vi "Recall Operating Mode.vi"(3 "error in":errorcluster, 4 "p1":i8, 5 "COM Port in":refnum<visa-resource-name>) -> (0 "error out":errorcluster, 1 "OK":bool, 2 "COM Port out":refnum<visa-resource-name>)   [LabVIEW 2013]
doc: "This command sets some bits of the operating mode through indexed presets.\n(Operating and bias level release, ACC/APC, analog/digital input releases and ICG activation)\n\nValid values for the parameter “p1” with PhoxX® lasers are:\no “0”: emission standby (the diode current source is set to 0)\no “1”: cw only – no modulation active\no “2”: digital modulated\no “3”: analog modulated\no “4”: digital and analog modulated\nAll other values will be refused.\n\nValid values for the parameter “p1” with LuxX® lasers are:\no “0”: emission standby (the diode current source is set to 0)\no “1”: ACC mode – no modulation active\no “2”: APC mode – no modulation active\no “3”: ACC mode – analog modulated\nAll other values will be refused.\n\nValid values for the parameter “p1” with LuxX+® and BrixX® lasers are:\no “0”: emission standby (the diode current source is set to 0)\no “1”: ACC mode – no modulation active\no “2”: APC mode – no modulation active\no “3”: ACC mode – digital modulated\no “4”: ACC mode – analog modulated\no “5”: ACC mode – digital and analog modulated\nAll other values will be refused.\n\nValid values for the parameter “p1” with LEDMOD.v2 are:\no “0”: emission standby (the diode current source is set to 0)\no “1”: cw only – no modulation active\no “2”: digital modulated\no “3”: analog modulated\no “4”: digital and analog modulated\no “5”: Internally PWM modulated - internal clock generator active (ICG)\no “6”: Internally PWM modulated - gated by external digital input\no “7”: Internally PWM modulated - externally modulated by analog input\no “8”: Internally PWM modulated - gated by digital input + externally modulated by analog input\nAll other values will be refused."
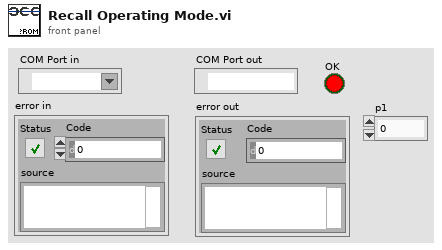
[diagram p1: front panel]
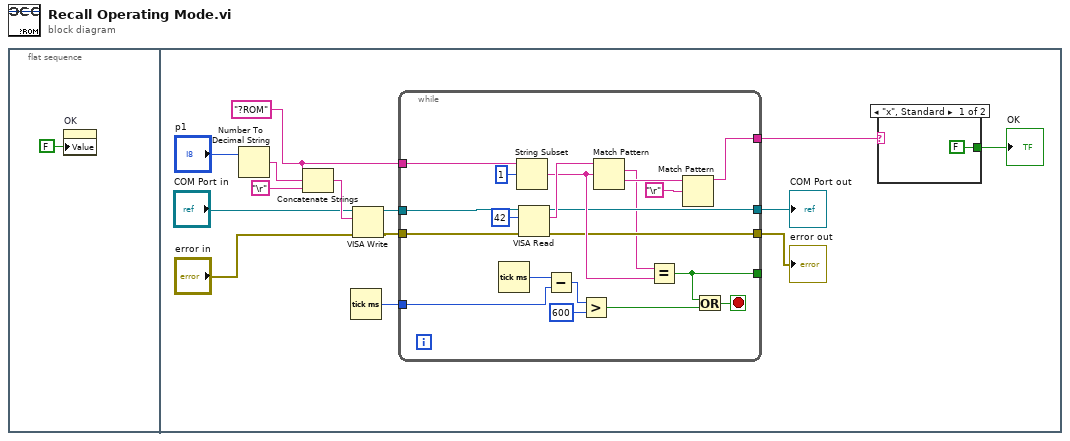
[diagram p0: block diagram]
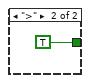
[diagram p2: hidden frame]
diagram:
  n1 = flat-sequence {
    frame #0 {
      n2 = property on="OK" class="Bool. (strikt)"("Value"=FALSE ("OK")) -> ()  [unwired: 2 in, 2 out]
    }
    frame #1 {
      w8 = "?ROM" ("Schreibpuffer")
      n3 = Number To Decimal String(number="p1") -> (decimal integer string=w2:string)  [unwired: 1 in]
      n4 = Concatenate Strings(w8, w2, "\r") -> (w13:string)
      n5 = Tick Count (ms)() -> (millisecond timer value=w7:u32)
      n6 = VISA Write(VISA resource name="COM Port in", write buffer=w13, error in (no error)="error in") -> (VISA resource name out=w10:refnum<visa-resource-name>, error out=w9:errorcluster)  [unwired: 1 out]
      n7 = while {
        tunnel: [w33] -> w15
        tunnel: [w32] -> w14
        tunnel: [w31] -> w6
        tunnel: [w27] -> _
        tunnel: w10 -> [w20]
        tunnel: w9 -> [w29]
        tunnel: w8 -> [w28]
        tunnel: w7 -> [w24]
        stop <- w26 stop-if-true
        n8 = Tick Count (ms)() -> (millisecond timer value=w25:u32)
        n9 = String Subset(string=w28, offset (0)=1 ("Offset (0)")) -> (substring=w34:string)  [unwired: 1 in]
        n10 = VISA Read(VISA resource name=w20, byte count=u32 42 ("Byte-Anzahl"), error in (no error)=w29) -> (VISA resource name out=w33:refnum<visa-resource-name>, read buffer=w36:string, error out=w32:errorcluster)  [unwired: 1 out]
        n11 = Subtract(x=w25, y=w24) -> (x-y=w23:u32)
        n12 = Greater?(x=w23, y=u32 600) -> (0:w21:bool)
        n13 = Match Pattern(string=w36, regular expression=w34) -> (match substring=w19:string, after substring=w30:string)  [unwired: 1 in, 2 out]
        n14 = Equal?(x=w19, y=w34) -> (x = y?=w27:bool)
        n15 = Match Pattern(string=w30, regular expression="\r") -> (before substring=w31:string)  [unwired: 1 in, 3 out]
        n16 = Or(x=w27, y=w21) -> (x .or. y?=w26:bool)
      }
      "COM Port out" <- w15
      "error out" <- w14
      n17 = case shown="\"x\", Standard" w6 {
        tunnel: [FALSE TRUE] -> w5
        frame "x", Default {
        }
        frame ">" {
        }
      }
      "OK" <- w5
    }
  }
